vi "PIDSetGains.vi"(0 "Refnum in":refnum<k20>, 1 "LegGains":T1={"Kp"=1200, "Ki"=0, "Kd"=800, "Kaw"=0, "Kff"=0}) -> (8 "PacketOut":u8[](array[numeric]))   [LabVIEW 2013]
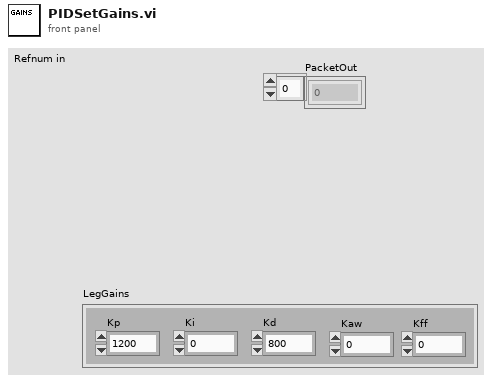
[diagram p1: front panel]
types:
  T1 = cluster{"Kp":u16, "Ki":u16, "Kd":u16, "Kaw":u16, "Kff":u16}
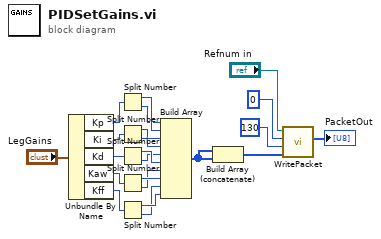
[diagram p0: block diagram]
diagram:
  n1 = Unbundle By Name("LegGains") -> ("Kp"=w5:u16, "Ki"=w4:u16, "Kd"=w3:u16, "Kaw"=w2:u16, "Kff"=w1:u16)
  n2 = Split Number(x=w5) -> (hi(x)=w19:u8, lo(x)=w18:u8)
  n3 = Split Number(x=w4) -> (hi(x)=w16:u8, lo(x)=w17:u8)
  n4 = Split Number(x=w3) -> (hi(x)=w15:u8, lo(x)=w14:u8)
  n5 = Split Number(x=w2) -> (hi(x)=w13:u8, lo(x)=w12:u8)
  n6 = Split Number(x=w1) -> (hi(x)=w11:u8, lo(x)=w10:u8)
  n7 = Build Array(w18, w19, w17, w16, w14, w15, w12, w13, w10, w11) -> (w9:u8[])
  n8 = Build Array (concatenate)(w9, w9) -> (w8:u8[])
  n9 = call "WritePacket.vi"("Payload"=w8, "Type"=u8 130, "Status"=u8 0, "Refnum in"="Refnum in") -> ("PacketOut"=→"PacketOut":u8[])  [unwired: 7 in]
